vi "just the pwm for exhaust.vi"() -> ()   [LabVIEW 2018]
uses:
  <vilib>/DAQmx/write.llb/DAQmx Write (Digital 1D Bool 1Chan 1Samp).vi
  <vilib>/DAQmx/write.llb/DAQmx Write (Digital 1D Bool NChan 1Samp 1Line).vi
  <vilib>/Waveform/DWDTOps.llb/DWDT Analog to Digital.vi
  <vilib>/Waveform/DWDTOps.llb/DWDT Digital to Boolean Array.vi
  <vilib>/DAQmx/create/channels.llb/DAQmx Create Channel (DO-Digital Output).vi
  <vilib>/DAQmx/miscellaneous.llb/DAQmx Fill In Error Info.vi
  <vilib>/measure/NI_MABase.lvlib
panel:
  out "?":bool
  in  "Exhaust Valve PWM  duty cycle (%)":dbl=50.0
  in  "stop":bool
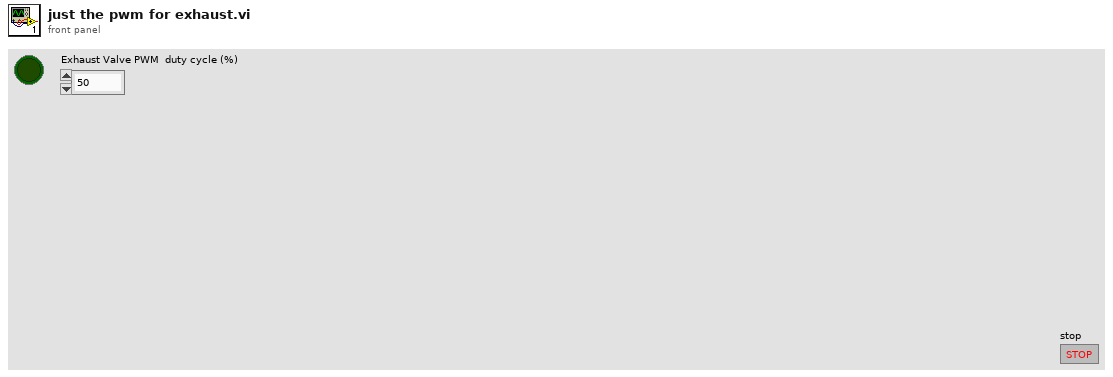
[diagram p1: front panel]
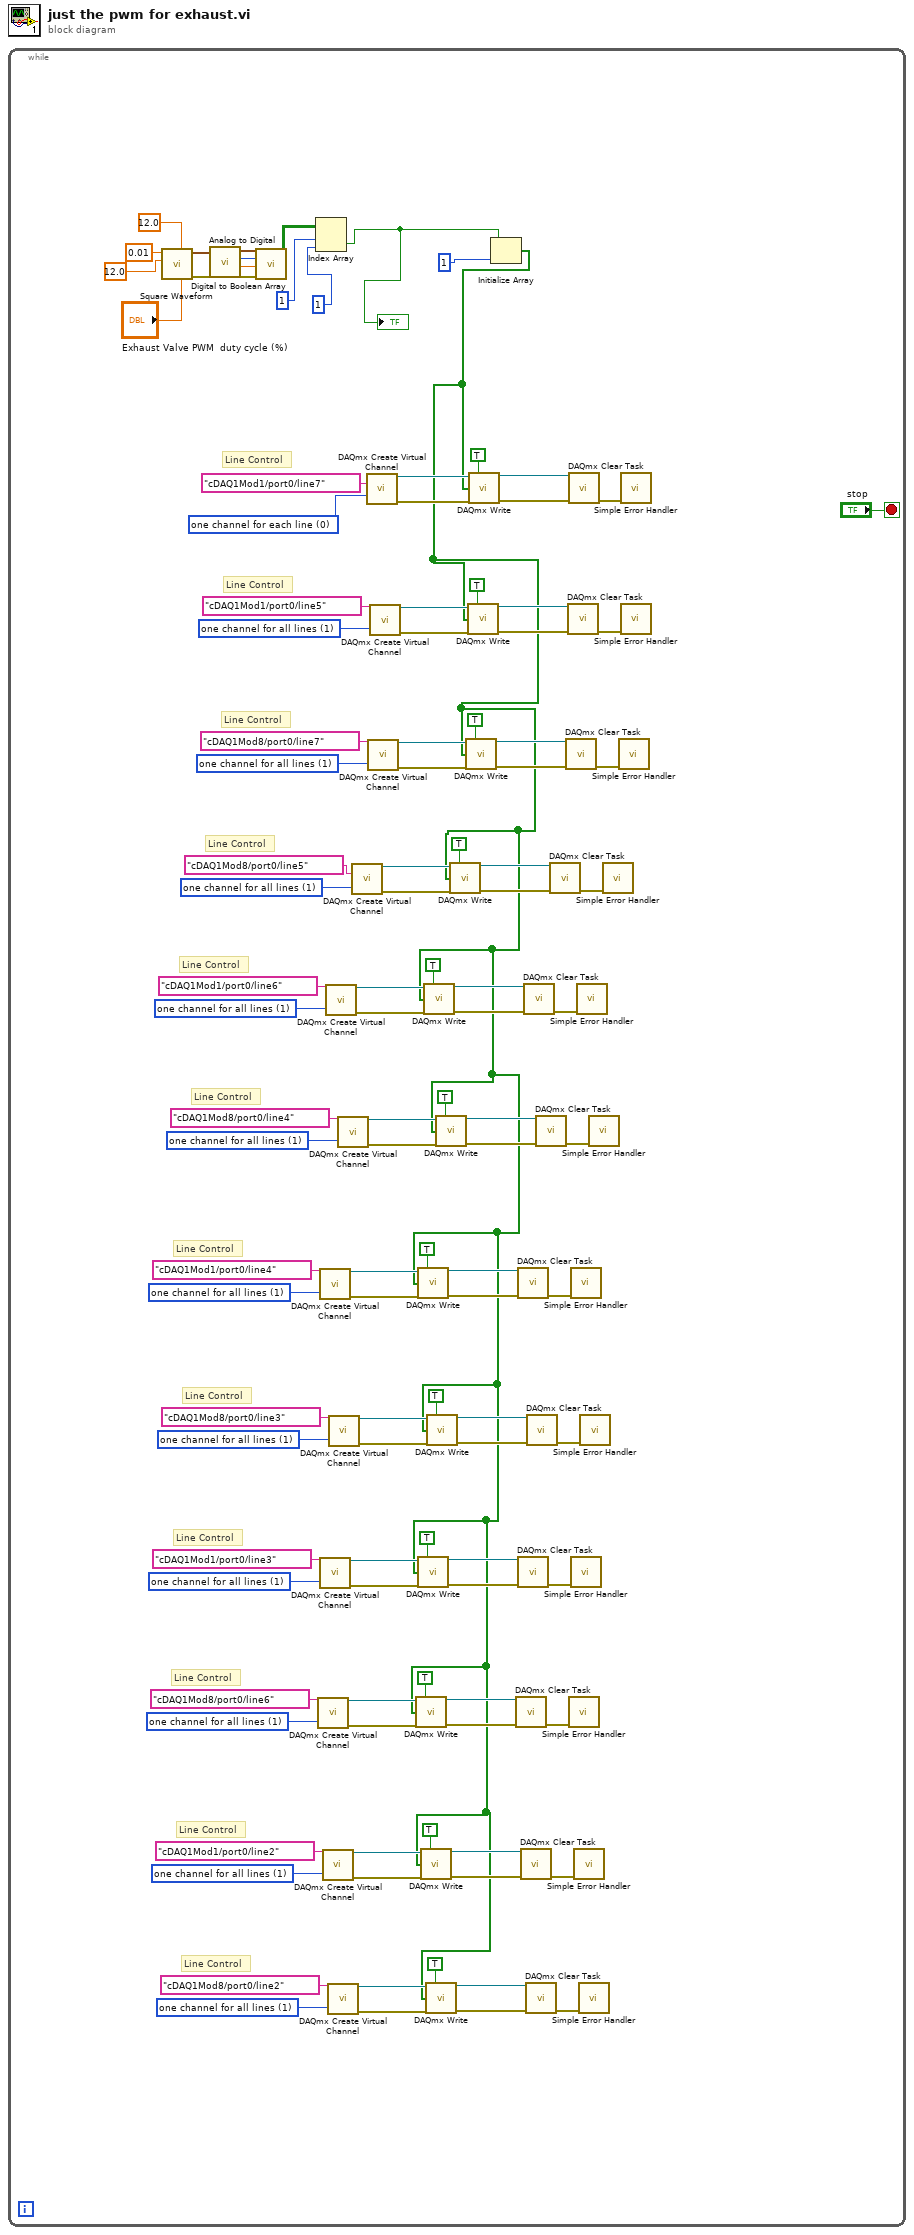
[diagram p0: block diagram]
diagram:
  n1 = while {
    stop <- "stop" stop-if-true
    w3 = 1 items=["one channel for each line", "one channel for all lines"] ("line grouping")
    w11 = 1 items=["one channel for each line", "one channel for all lines"] ("line grouping")
    w19 = 1 items=["one channel for each line", "one channel for all lines"] ("line grouping")
    w27 = 1 items=["one channel for each line", "one channel for all lines"] ("line grouping")
    w35 = 1 items=["one channel for each line", "one channel for all lines"] ("line grouping")
    w43 = 1 items=["one channel for each line", "one channel for all lines"] ("line grouping")
    w51 = 1 items=["one channel for each line", "one channel for all lines"] ("line grouping")
    w59 = 1 items=["one channel for each line", "one channel for all lines"] ("line grouping")
    w67 = 1 items=["one channel for each line", "one channel for all lines"] ("line grouping")
    w75 = 1 items=["one channel for each line", "one channel for all lines"] ("line grouping")
    w83 = 0 items=["one channel for each line", "one channel for all lines"] ("line grouping")
    w86 = 1 items=["one channel for each line", "one channel for all lines"] ("line grouping")
    # "Line Control"
    # "Line Control"
    # "Line Control"
    # "Line Control"
    # "Line Control"
    # "Line Control"
    # "Line Control"
    # "Line Control"
    # "Line Control"
    # "Line Control"
    # "Line Control"
    # "Line Control"
    n2 = call <vilib>:"Square Waveform.vi"("duty cycle (%)"="Exhaust Valve PWM  duty cycle (%)", "offset"=12.0, "amplitude"=12.0, "frequency"=0.01) -> ("error out"=w106:errorcluster, "signal out"=w99:waveform(dbl))  [unwired: 6 in]
    n3 = call-poly <vilib>:"Analog to Digital.vi"("error in (no error)"=w106, "analog waveform"=w99) -> ("error out"=w108:errorcluster, "full-scale range (out)"=w109:dbl, "resolution (out)"=w110:i32, "digital waveform"=w107:digitalwaveform)  [unwired: 6 in]
    n4 = call-poly <vilib>:"Digital to Boolean Array.vi"("error in (no error)"=w108, "mode"=w109, "response on error"=w110, "digital waveform"=w107) -> ("boolean array"=w112:bool[][])  [unwired: 6 in, 1 out]
    n5 = Index Array(array=w112, index (row)=1, index (col)=1 ("disabled index (col)")) -> (element=w82:bool)
    "?" <- w82
    n6 = call-poly <vilib>:"DAQmx Create Virtual Channel.vi"("lines"=tag "cDAQ1Mod8/port0/line6", "line grouping"=w19) -> ("task out"=w21:refnum<k21>, "error out"=w20:errorcluster)  [unwired: 12 in]
    n7 = call-poly <vilib>:"DAQmx Create Virtual Channel.vi"("lines"=tag "cDAQ1Mod1/port0/line4", "line grouping"=w43) -> ("task out"=w45:refnum<k21>, "error out"=w44:errorcluster)  [unwired: 12 in]
    n8 = call-poly <vilib>:"DAQmx Create Virtual Channel.vi"("lines"=tag "cDAQ1Mod1/port0/line3", "line grouping"=w27) -> ("task out"=w29:refnum<k21>, "error out"=w28:errorcluster)  [unwired: 12 in]
    n9 = call-poly <vilib>:"DAQmx Create Virtual Channel.vi"("lines"=tag "cDAQ1Mod1/port0/line2", "line grouping"=w11) -> ("task out"=w13:refnum<k21>, "error out"=w12:errorcluster)  [unwired: 12 in]
    n10 = call-poly <vilib>:"DAQmx Create Virtual Channel.vi"("lines"=tag "cDAQ1Mod1/port0/line6", "line grouping"=w59) -> ("task out"=w61:refnum<k21>, "error out"=w60:errorcluster)  [unwired: 12 in]
    n11 = call-poly <vilib>:"DAQmx Create Virtual Channel.vi"("lines"=tag "cDAQ1Mod8/port0/line2", "line grouping"=w3) -> ("task out"=w5:refnum<k21>, "error out"=w4:errorcluster)  [unwired: 12 in]
    n12 = call-poly <vilib>:"DAQmx Create Virtual Channel.vi"("lines"=tag "cDAQ1Mod8/port0/line3", "line grouping"=w35) -> ("task out"=w37:refnum<k21>, "error out"=w36:errorcluster)  [unwired: 12 in]
    n13 = call-poly <vilib>:"DAQmx Create Virtual Channel.vi"("lines"=tag "cDAQ1Mod8/port0/line4", "line grouping"=w51) -> ("task out"=w53:refnum<k21>, "error out"=w52:errorcluster)  [unwired: 12 in]
    n14 = call-poly <vilib>:"DAQmx Create Virtual Channel.vi"("lines"=tag "cDAQ1Mod8/port0/line5", "line grouping"=w67) -> ("task out"=w71:refnum<k21>, "error out"=w72:errorcluster)  [unwired: 12 in]
    n15 = call-poly <vilib>:"DAQmx Create Virtual Channel.vi"("lines"=tag "cDAQ1Mod1/port0/line7", "line grouping"=w83) -> ("task out"=w96:refnum<k21>, "error out"=w95:errorcluster)  [unwired: 12 in]
    n16 = call-poly <vilib>:"DAQmx Create Virtual Channel.vi"("lines"=tag "cDAQ1Mod8/port0/line7", "line grouping"=w75) -> ("task out"=w77:refnum<k21>, "error out"=w76:errorcluster)  [unwired: 12 in]
    n17 = call-poly <vilib>:"DAQmx Create Virtual Channel.vi"("lines"=tag "cDAQ1Mod1/port0/line5", "line grouping"=w86) -> ("task out"=w88:refnum<k21>, "error out"=w87:errorcluster)  [unwired: 12 in]
    n18 = Initialize Array(w82, 1 ("dimension size")) -> (w1:bool[])
    n19 = call-poly <vilib>:"DAQmx Write.vi"("task/channels in"=w21, "auto start"=TRUE, "data"=w1, "error in"=w20) -> ("task out"=w23:refnum<k21>, "error out"=w24:errorcluster)  [unwired: 9 in, 1 out]
    n20 = call-poly <vilib>:"DAQmx Write.vi"("task/channels in"=w45, "auto start"=TRUE, "data"=w1, "error in"=w44) -> ("task out"=w47:refnum<k21>, "error out"=w48:errorcluster)  [unwired: 9 in, 1 out]
    n21 = call-poly <vilib>:"DAQmx Write.vi"("task/channels in"=w29, "auto start"=TRUE, "data"=w1, "error in"=w28) -> ("task out"=w31:refnum<k21>, "error out"=w32:errorcluster)  [unwired: 9 in, 1 out]
    n22 = call-poly <vilib>:"DAQmx Write.vi"("task/channels in"=w13, "auto start"=TRUE, "data"=w1, "error in"=w12) -> ("task out"=w15:refnum<k21>, "error out"=w16:errorcluster)  [unwired: 9 in, 1 out]
    n23 = call-poly <vilib>:"DAQmx Write.vi"("task/channels in"=w61, "auto start"=TRUE, "data"=w1, "error in"=w60) -> ("task out"=w63:refnum<k21>, "error out"=w64:errorcluster)  [unwired: 9 in, 1 out]
    n24 = call-poly <vilib>:"DAQmx Write.vi"("task/channels in"=w5, "auto start"=TRUE, "data"=w1, "error in"=w4) -> ("task out"=w7:refnum<k21>, "error out"=w8:errorcluster)  [unwired: 9 in, 1 out]
    n25 = call-poly <vilib>:"DAQmx Write.vi"("task/channels in"=w37, "auto start"=TRUE, "data"=w1, "error in"=w36) -> ("task out"=w39:refnum<k21>, "error out"=w40:errorcluster)  [unwired: 9 in, 1 out]
    n26 = call-poly <vilib>:"DAQmx Write.vi"("task/channels in"=w53, "auto start"=TRUE, "data"=w1, "error in"=w52) -> ("task out"=w55:refnum<k21>, "error out"=w56:errorcluster)  [unwired: 9 in, 1 out]
    n27 = call-poly <vilib>:"DAQmx Write.vi"("task/channels in"=w71, "auto start"=TRUE, "data"=w1, "error in"=w72) -> ("task out"=w70:refnum<k21>, "error out"=w69:errorcluster)  [unwired: 9 in, 1 out]
    n28 = call-poly <vilib>:"DAQmx Write.vi"("task/channels in"=w77, "auto start"=TRUE, "data"=w1, "error in"=w76) -> ("task out"=w79:refnum<k21>, "error out"=w80:errorcluster)  [unwired: 9 in, 1 out]
    n29 = call-poly <vilib>:"DAQmx Write.vi"("task/channels in"=w88, "auto start"=TRUE, "data"=w1, "error in"=w87) -> ("task out"=w90:refnum<k21>, "error out"=w91:errorcluster)  [unwired: 9 in, 1 out]
    n30 = call-poly <vilib>:"DAQmx Write.vi"("task/channels in"=w96, "auto start"=TRUE, "data"=w1, "error in"=w95) -> ("task out"=w93:refnum<k21>, "error out"=w92:errorcluster)  [unwired: 9 in, 1 out]
    n31 = call <vilib>:"DAQmx Clear Task.vi"("task in"=w23, "error in"=w24) -> ("error out"=w18:errorcluster)  [unwired: 13 in]
    n32 = call <vilib>:"DAQmx Clear Task.vi"("task in"=w47, "error in"=w48) -> ("error out"=w42:errorcluster)  [unwired: 13 in]
    n33 = call <vilib>:"DAQmx Clear Task.vi"("task in"=w31, "error in"=w32) -> ("error out"=w26:errorcluster)  [unwired: 13 in]
    n34 = call <vilib>:"DAQmx Clear Task.vi"("task in"=w15, "error in"=w16) -> ("error out"=w10:errorcluster)  [unwired: 13 in]
    n35 = call <vilib>:"DAQmx Clear Task.vi"("task in"=w63, "error in"=w64) -> ("error out"=w58:errorcluster)  [unwired: 13 in]
    n36 = call <vilib>:"DAQmx Clear Task.vi"("task in"=w7, "error in"=w8) -> ("error out"=w2:errorcluster)  [unwired: 13 in]
    n37 = call <vilib>:"DAQmx Clear Task.vi"("task in"=w39, "error in"=w40) -> ("error out"=w34:errorcluster)  [unwired: 13 in]
    n38 = call <vilib>:"DAQmx Clear Task.vi"("task in"=w55, "error in"=w56) -> ("error out"=w50:errorcluster)  [unwired: 13 in]
    n39 = call <vilib>:"DAQmx Clear Task.vi"("task in"=w70, "error in"=w69) -> ("error out"=w73:errorcluster)  [unwired: 13 in]
    n40 = call <vilib>:"DAQmx Clear Task.vi"("task in"=w79, "error in"=w80) -> ("error out"=w74:errorcluster)  [unwired: 13 in]
    n41 = call <vilib>:"DAQmx Clear Task.vi"("task in"=w90, "error in"=w91) -> ("error out"=w84:errorcluster)  [unwired: 13 in]
    n42 = call <vilib>:"DAQmx Clear Task.vi"("task in"=w93, "error in"=w92) -> ("error out"=w85:errorcluster)  [unwired: 13 in]
    n43 = call <vilib>:"Simple Error Handler.vi"("error in (no error)"=w18) -> ()  [unwired: 4 in, 5 out]
    n44 = call <vilib>:"Simple Error Handler.vi"("error in (no error)"=w42) -> ()  [unwired: 4 in, 5 out]
    n45 = call <vilib>:"Simple Error Handler.vi"("error in (no error)"=w26) -> ()  [unwired: 4 in, 5 out]
    n46 = call <vilib>:"Simple Error Handler.vi"("error in (no error)"=w10) -> ()  [unwired: 4 in, 5 out]
    n47 = call <vilib>:"Simple Error Handler.vi"("error in (no error)"=w58) -> ()  [unwired: 4 in, 5 out]
    n48 = call <vilib>:"Simple Error Handler.vi"("error in (no error)"=w2) -> ()  [unwired: 4 in, 5 out]
    n49 = call <vilib>:"Simple Error Handler.vi"("error in (no error)"=w34) -> ()  [unwired: 4 in, 5 out]
    n50 = call <vilib>:"Simple Error Handler.vi"("error in (no error)"=w50) -> ()  [unwired: 4 in, 5 out]
    n51 = call <vilib>:"Simple Error Handler.vi"("error in (no error)"=w73) -> ()  [unwired: 4 in, 5 out]
    n52 = call <vilib>:"Simple Error Handler.vi"("error in (no error)"=w74) -> ()  [unwired: 4 in, 5 out]
    n53 = call <vilib>:"Simple Error Handler.vi"("error in (no error)"=w85) -> ()  [unwired: 4 in, 5 out]
    n54 = call <vilib>:"Simple Error Handler.vi"("error in (no error)"=w84) -> ()  [unwired: 4 in, 5 out]
  }
